vi "Home Filter Wheel.vi"(8 "error in (no error)":errorcluster, 10 "Motor":i32, 11 "FW Arduino Control in":refnum<class "FW Arduino Control.lvclass">) -> (0 "error out":errorcluster, 1 "Success":bool, 2 "Log":string, 3 "FW Arduino Control out":refnum<class "FW Arduino Control.lvclass">)   [LabVIEW 2024, in "FW Arduino Control.lvclass"]
uses:
  FW Arduino Control.lvclass
  Filter Wheel Object/Filter Wheel.lvclass
  FW Arduino Control.lvclass/FW Arduino Control.ctl
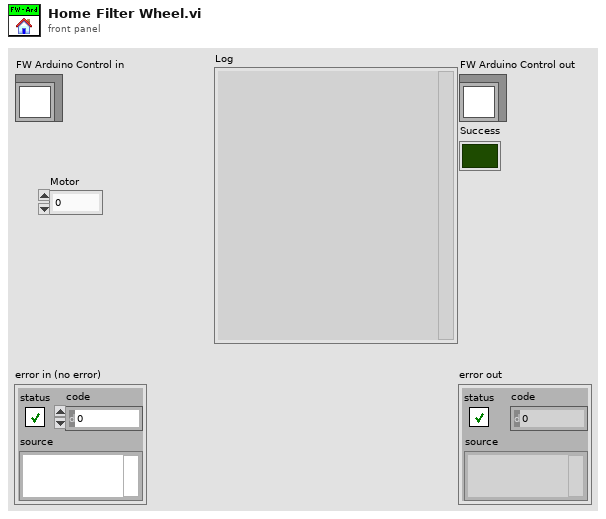
[diagram p1: front panel]
types:
  T1 = typedef "Filter Wheel Arduino Homing cluster.ctl" = cluster{"Direction":bool, "Speed":i32, "Accel":i32, "Error Cnts":i32, "Homing Delta":i32}
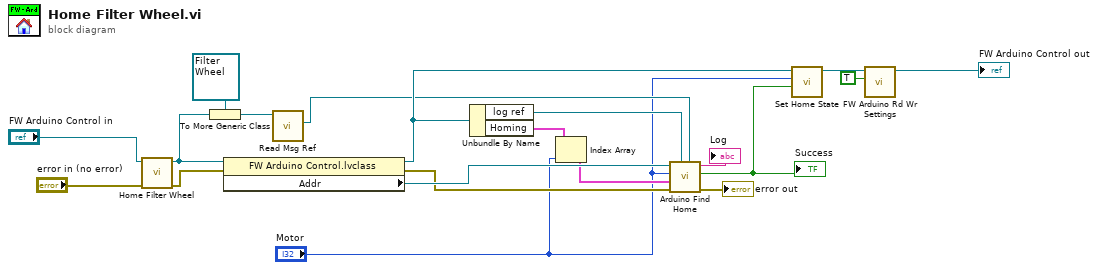
[diagram p0: block diagram]
diagram:
  n1 = call-parent "Home Filter Wheel.vi"("error in (no error)"="error in (no error)", "Filter Wheel in"="FW Arduino Control in") -> ("error out"=w18:errorcluster, "Filter Wheel out"=w6:refnum<class "FW Arduino Control.lvclass">)  [unwired: 6 in, 2 out]
  n2 = To More Generic Class(target class=refnum<class "Filter Wheel.lvclass"> refnum ("Filter Wheel.lvclass"), reference=w6) -> (generic class reference=w4:refnum<class "Filter Wheel.lvclass">)
  n3 = property class="FW Arduino Control.lvclass"(reference=w6, error in=w18) -> (reference out=w10:refnum<class "FW Arduino Control.lvclass">, error out=w16:errorcluster, "Addr"=w17:refnum<visa-resource-name>)
  n4 = call-dynamic "Read Msg Ref.vi"("Filter Wheel in"=w4) -> ("Msg Ref"=w3:refnum<vi>)  [unwired: 8 in, 2 out]
  n5 = Unbundle By Name(w10) -> ("log ref"=w11:refnum<file>, "Homing"=w14:T1[])
  n6 = Index Array(array=w14, index="Motor") -> (element=w2:T1)
  n7 = call "Arduino Find Home.vi"("Msg Ref"=w3, "log ref"=w11, "error in"=w16, "Homing Parameters"=w2, "Motor"="Motor", "Addr"=w17) -> ("error out"=→"error out":errorcluster, "Success"=w12:bool, "Log"=→"Log":string)  [unwired: 3 in]
  "Success" <- w12
  n8 = call "Set Home State.vi"("Home?"=w12, "Motor"="Motor", "Filter Wheel in"=w10) -> ("Filter Wheel out"=w9:refnum<class "FW Arduino Control.lvclass">)  [unwired: 7 in, 1 out]
  n9 = call "FW Arduino Rd Wr Settings.vi"("Write? (F:Read)"=TRUE, "Settings"=w9) -> ("Settings"=→"FW Arduino Control out":refnum<class "FW Arduino Control.lvclass">)  [unwired: 8 in, 1 out]
